vi "MapObjectID.vi"(5 "error in (no error)":errorcluster) -> (15 "proxy ID":u32[](array[numeric]), 16 "remote ID":u32[](array[numeric]), 19 "error out":errorcluster)   [LabVIEW 2017, in "G#RemoteProxy.lvclass"]
doc: "Maps the remote object id with the proxy object id."
uses:
  G#RemoteProxy.lvclass
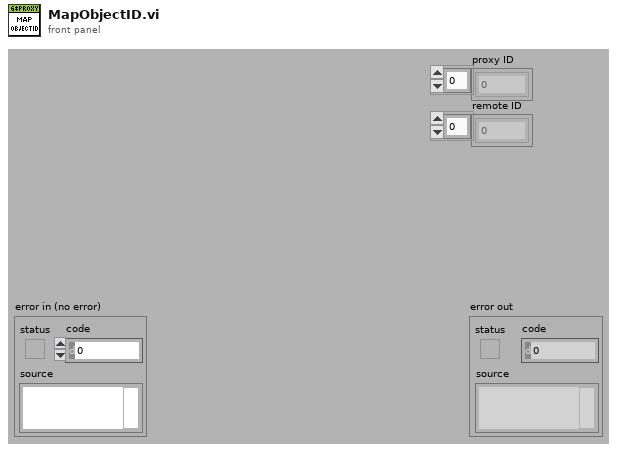
[diagram p1: front panel]
types:
  T1 = typedef "G#RemoteProxy.lvclass/ClassAttributesProxy.ctl" = cluster{"NoActiveProject":bool, "FullClassNames":string[], "FullClassPaths":path[], "RemoteRefs":refnum<class "G#Object.lvclass">[], "ProxyRefs":refnum<class "G#RemoteProxy.lvclass">[], "RemoteClassName":string[], "ProxyClassRefs":refnum<class "G#RemoteProxy.lvclass">[]}
  T2 = typedef "G#RemoteProxy.lvclass/ObjectAttributesProxy.ctl" = cluster{"class hierarchy":T3[], "class name":string, "lvlib hierarchy":string[], "full class name":string, "id":u32, "owner":string, "RemoteRef":refnum<class "G#Object.lvclass">, "object name":string, "attributes":variant[], "connection ID":refnum<k5>, "address":u32, "occurrence":refnum<k4>, "ProxyClassRef":refnum<class "G#RemoteProxy.lvclass">, "InMemory?":bool, "ToString":string}
  T3 = typedef "G#Object.lvclass/G#Object_ClassHierarchy.ctl" = cluster{"ClassName":string, "FullClassName":string, "ClassPath":path, "IsLeaf":bool}
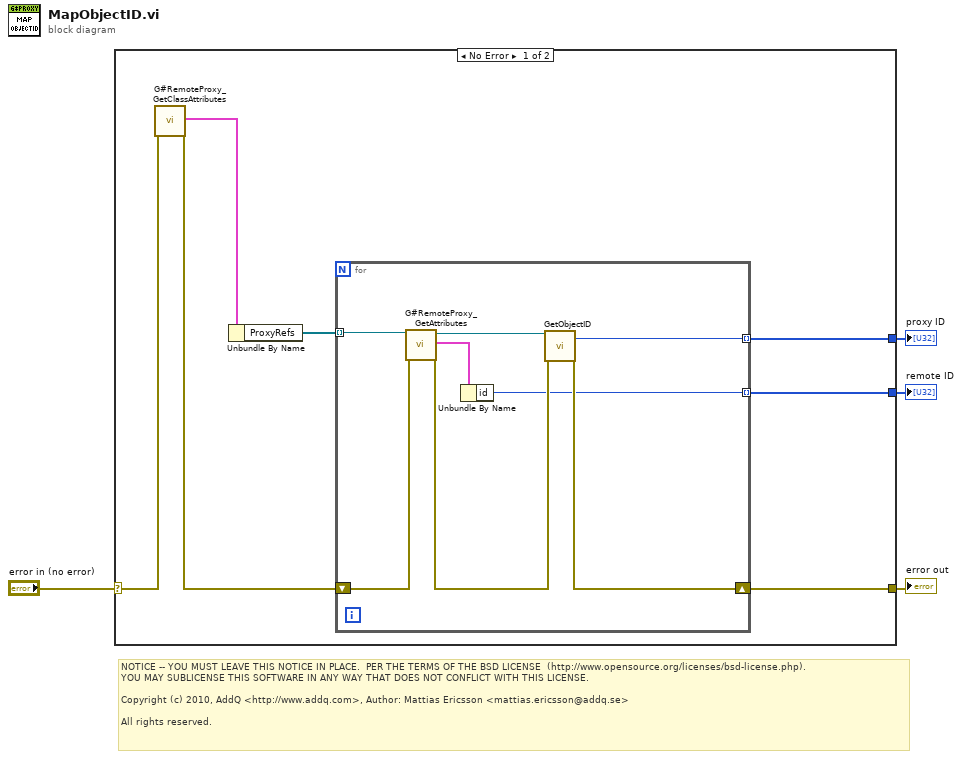
[diagram p0: block diagram]
diagram:
  # "NOTICE -- YOU MUST LEAVE THIS NOTICE IN PLACE.  PER THE TERMS OF THE BSD LICENSE  (http://www.opensource.org/licenses/bsd-license.php).\nYOU MAY SUBLICENSE THIS SOFTWARE IN ANY WAY THAT DOES NOT CONFLICT WITH THIS LICENSE.\n\nCopyright (c) 2010, AddQ <http://www.addq.com>, Author: Mattias Ericsson <mattias.ericsson@addq.se>\n\nAll rights reserved."
  n1 = case shown="No Error" "error in (no error)" {
    selector: "error in (no error)" -> [w11 w20]
    tunnel: [w5 w20] -> w3
    tunnel: [w7 _] -> w2
    tunnel: [w6 _] -> w1
    frame No Error {
      n2 = call "G#RemoteProxy_GetClassAttributes.vi"("error in (no error)"=w11) -> ("class attributes"=w10:T1, "error out"=w9:errorcluster)  [unwired: 15 in, 2 out]
      n3 = Unbundle By Name(w10) -> ("ProxyRefs"=w8:refnum<class "G#RemoteProxy.lvclass">[])
      n4 = for {
        shift-right: [w14] -> w5
        shift-left: w9 -> [w18]
        tunnel: w8 -> [w19] mode=indexing
        tunnel: [w13] -> w7 mode=indexing
        tunnel: [w12] -> w6 mode=indexing
        n5 = call "G#RemoteProxy_GetAttributes.vi"("reference in"=w19, "error in (no error)"=w18) -> ("reference out"=w16:refnum<class "G#RemoteProxy.lvclass">, "attributes"=w17:T2, "error out"=w15:errorcluster)  [unwired: 14 in, 1 out]
        n6 = Unbundle By Name(w17) -> ("id"=w12:u32)
        n7 = call-dynamic "GetObjectID.vi"("reference in"=w16, "error in (no error)"=w15) -> ("object ID"=w13:u32, "error out"=w14:errorcluster)  [unwired: 15 in, 1 out]
      }
    }
    frame Error {
    }
  }
  "error out" <- w3
  "proxy ID" <- w2
  "remote ID" <- w1
